vi "Equi-Ripple HighPass (CDB).vi"(0 "# of taps":i32=33, 1 "stop freq":dbl=0.2 format="%0.2f", 2 "high freq":dbl=0.25 format="%0.2f", 3 "sampling freq: fs":dbl=1.0 format="%0.2f", 5 "X":cdb[](array[numeric])) -> (4 "error":i32, 7 "Filtered X":cdb[](array[numeric]))   [LabVIEW 2017, in "NI_AALBase.lvlib"]
doc: "Generates a highpass FIR filter with equi-ripple characteristics using the Parks-McClellan algorithm and the <B># of taps</B>, <B>stop freq</B>, <B>high freq</B>, and <B>sampling freq: fs</B>. The Equi-Ripple HighPass VI then applies a linear-phase, highpass filter to the input sequence <B>X</B> using the Convolution VI to obtain <B>Filtered X</B>. Wire data to the <B>X</B> input to determine the polymorphic instance to use or manually select the instance."
uses:
  <vilib>/Analysis/NI_AALBase.lvlib
  <vilib>/Analysis/2dsp.llb/1D Convolution (DBL).vi
  <vilib>/Analysis/NI_AALPro.lvlib
panel:
  # "Equi-Ripple\n Highpass FIR Filter"
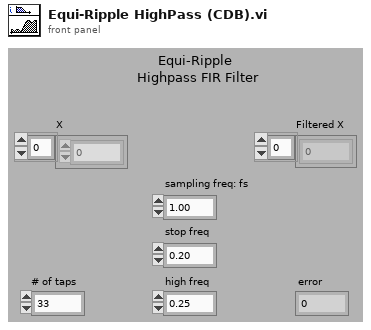
[diagram p1: front panel]
types:
  T1 = cluster{"Amplitude":dbl, "DC":dbl, "stop freq":dbl, "Weight":dbl}
  T2 = cluster{"Amplitude":dbl, "high freq":dbl, dbl, "Weight":dbl}
  T3 = cluster{"Amplitude":dbl, "high freq":dbl, "stop freq":dbl, "Weight":dbl}[]
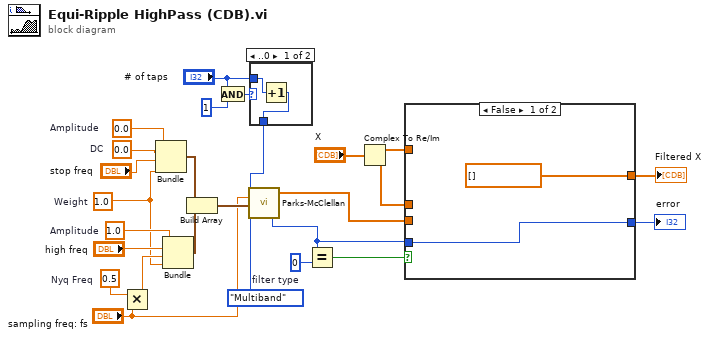
[diagram p0: block diagram]
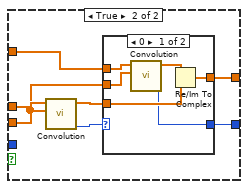
[diagram p2: hidden frame]
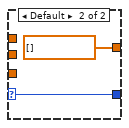
[diagram p3: hidden frame]
diagram:
  w16 = enum32{"Multiband", "Differentiator", "Hilbert"}."Multiband"  # filter type
  w11 = 1.0  # Weight
  w24 = 0.5  # Nyq Freq
  w12 = 1.0  # Amplitude
  w9 = 0.0  # DC
  w10 = 0.0  # Amplitude
  n1 = Multiply(x=w24, y="sampling freq: fs") -> (x*y=w23:dbl)
  n2 = Bundle("Amplitude"=w10, "DC"=w9, "stop freq"="stop freq", "Weight"=w11) -> (w22:T1)  [unwired: 1 in]
  n3 = Bundle("Amplitude"=w12, "high freq"="high freq", w23, "Weight"=w11) -> (w21:T2)  [unwired: 1 in]
  n4 = Build Array(w22, w21) -> (w15:T3)
  n5 = And(x="# of taps", y=1) -> (x .and. y?=w19:i32)
  n6 = case shown="..0" w19 {
    tunnel: "# of taps" -> [w28 w29]
    tunnel: [w27 w29] -> w17
    frame ..0 {
      n7 = Increment(x=w28) -> (x+1=w27:i32)
    }
    frame 1.. {
    }
  }
  n8 = call <vilib>:"Parks-McClellan.vi"("filter type"=w16, "Band Parameters"=w15, "sampling freq: fs"="sampling freq: fs", "# of taps"=w17) -> ("error"=w3:i32, "h"=w5:dbl[])  [unwired: 1 out]
  n9 = Equal?(x=w3, y=0) -> (x = y?=w4:bool)
  n10 = Complex To Re/Im(x + iy="X") -> (x=w7:dbl[], y=w6:dbl[])
  n11 = case shown="False" w4 {
    tunnel: w3 -> [w31 _]
    tunnel: [w31 w32] -> w1
    tunnel: [cdb[] [] ("empty array") w34] -> w2
    tunnel: w6 -> [_ w38]
    tunnel: w5 -> [_ w35]
    tunnel: w7 -> [_ w36]
    frame False {
    }
    frame True {
      n12 = call-poly <vilib>:"Convolution.vi"("Y"=w35, "X"=w38) -> ("error"=w37:i32, "X * Y"=w33:dbl[])  [unwired: 8 in]
      n13 = case shown="0" w37 {
        selector: w37 -> [_ w45]
        tunnel: w36 -> [w44 _]
        tunnel: w35 -> [w43 _]
        tunnel: [w41 cdb[] [] ("empty array")] -> w34
        tunnel: w33 -> [w42 _]
        tunnel: [w40 w45] -> w32
        frame 0 {
          n14 = call-poly <vilib>:"Convolution.vi"("Y"=w43, "X"=w44) -> ("error"=w40:i32, "X * Y"=w39:dbl[])  [unwired: 8 in]
          n15 = Re/Im To Complex(1:w42, 2:w39) -> (0:w41:cdb[])
        }
        frame Default {
        }
      }
    }
  }
  "Filtered X" <- w2
  "error" <- w1
